vi "niRFUtil WFM Average (real wfm).vi"(0 "Waveform In":T2 {"y" min=0 max=127 format="%.2f"; "dx" format="%^.2e"; "x0" format="%^.2e"}, 5 "Average Mode":enum16{"Exponential", "Repeat"}(ring), 7 "Average Method":T1, 12 "Reset?":bool=TRUE, 13 "Initialize?":bool=TRUE) -> (4 "Average Out":T2 {"y" min=0 max=127 format="%.2f"; "dx" format="%^.2e"; "x0" format="%^.2e"})   [LabVIEW 2015, in "niRFUtil.lvlib"]
doc: "(c) Copyright 2006, National Instruments, Inc. This VI may not be duplicated, sold, or distributed without written consent from National Instruments."
uses:
  niRFUtil.lvlib
  Includes/niRFUtil INC Real Waveform.ctl
  Includes/niRFUtil INC Real Array.ctl
  Includes/niRFUtil INC Average Methods.ctl
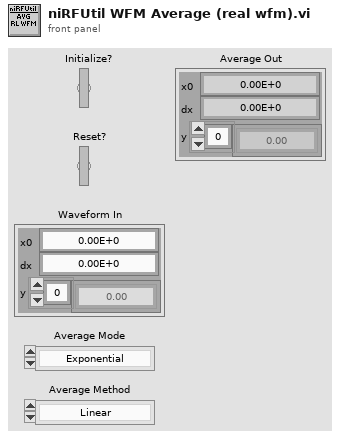
[diagram p1: front panel]
types:
  T1 = typedef "niRFUtil.lvlib/niRFUtil INC Average Methods.ctl" = enum16{"Linear", "Log", "Root", "Max", "Min", "MinMax"}
  T2 = typedef "niRFUtil.lvlib/niRFUtil INC Real Waveform.ctl" = cluster{"x0":dbl, "dx":dbl, "y":T3}
  T3 = typedef "niRFUtil.lvlib/niRFUtil INC Real Array.ctl" = sgl[]
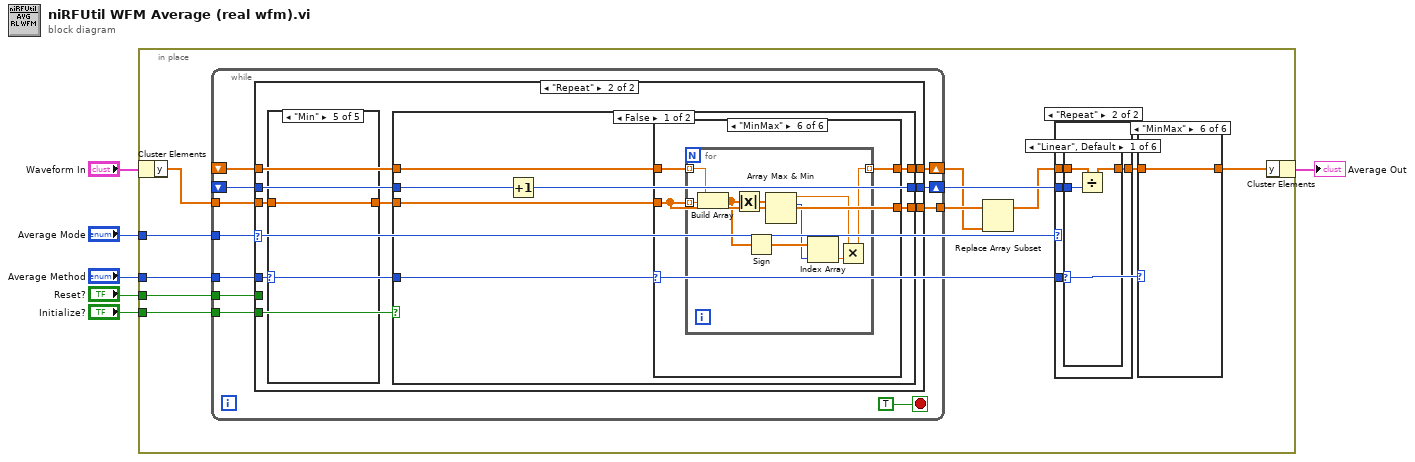
[diagram p0: block diagram]
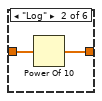
[diagram p3: hidden frame]
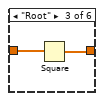
[diagram p4: hidden frame]
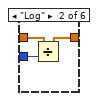
[diagram p8: hidden frame]
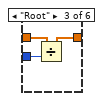
[diagram p9: hidden frame]
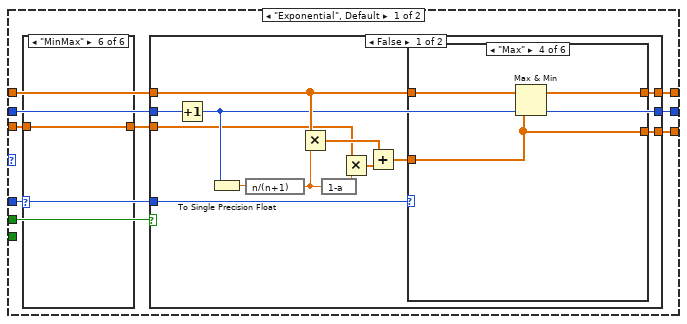
[diagram p13: hidden frame]
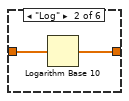
[diagram p15: hidden frame]
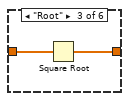
[diagram p16: hidden frame]
diagram:
  n1 = in-place {
    in-place-border: "Average Mode" -> [w16]
    in-place-border: "Average Method" -> [w15]
    in-place-border: "Reset?" -> [w14]
    in-place-border: "Initialize?" -> [w13]
    n2 = in-place-cluster #1("Waveform In") -> ("y"=w11:T3)
    n3 = while {
      shift-right: [w50] -> w8
      shift-left: _ -> [w47]
      tunnel: w16 -> [w52]
      tunnel: w14 -> [w51]
      tunnel: w11 -> [w49]
      shift-right: [w48] -> w17
      shift-left: _ -> [w46]
      tunnel: w15 -> [w45]
      tunnel: w13 -> [w44]
      tunnel: [w43] -> w9
      stop <- TRUE stop-if-true
      n4 = case shown="\"Repeat\"" w52 {
        tunnel: w51 -> [w59 _]
        tunnel: [w62 w115] -> w50
        tunnel: w49 -> [w57 w110]
        tunnel: [w58 w112] -> w48
        tunnel: w47 -> [w61 w114]
        tunnel: w46 -> [w60 w113]
        tunnel: w45 -> [w55 w108]
        tunnel: w44 -> [_ w111]
        tunnel: [w54 w107] -> w43
        frame "Exponential", Default {
          n5 = case shown="\"MinMax\"" w55 {
            tunnel: w57 -> [w63 w65 w67 w68 w69 w70]
            tunnel: [w63 w64 w66 w68 w69 w70] -> w56
            frame "Linear", Default {
            }
            frame "Log" {
              n6 = Logarithm Base 10(1:w65) -> (0:w64:T3)
            }
            frame "Root" {
              n7 = Square Root(x=w67) -> (sqrt(x)=w66:T3)
            }
            frame "Max" {
            }
            frame "Min" {
            }
            frame "MinMax" {
            }
          }
          n8 = case shown="False" w59 {
            tunnel: w56 -> [w72 w105]
            tunnel: [w78 w105] -> w62
            tunnel: w61 -> [w76 _]
            tunnel: w60 -> [w75 _]
            tunnel: [w74 1] -> w58
            tunnel: w55 -> [w73 _]
            tunnel: [w71 w105] -> w54
            frame False {
              n9 = Increment(x=w75) -> (x+1=w74:i32)
              n10 = To Single Precision Float(number=w74) -> (single precision float=w83:sgl)
              n11 = expression code="n/(n+1)"(w83) -> (w82:sgl)
              n12 = Multiply(x=w76, y=w82) -> (x*y=w79:T3)
              n13 = expression code="1-a"(w82) -> (w81:sgl)
              n14 = Multiply(x=w72, y=w81) -> (x*y=w80:T3)
              n15 = Add(x=w79, y=w80) -> (x+y=w77:T3)
              n16 = case shown="\"Max\"" w73 {
                tunnel: [w84 w85 w86 w88 w91 w94] -> w78
                tunnel: w77 -> [w84 w85 w86 w87 w90 w93]
                tunnel: w76 -> [_ _ _ w89 w92 w95]
                tunnel: [w84 w85 w86 w87 w90 w93] -> w71
                frame "Linear", Default {
                }
                frame "Log" {
                }
                frame "Root" {
                }
                frame "Max" {
                  n17 = Max & Min(x=w89, y=w87) -> (max(x,y)=w88:T3)  [unwired: 1 out]
                }
                frame "Min" {
                  n18 = Max & Min(x=w92, y=w90) -> (min(x,y)=w91:T3)  [unwired: 1 out]
                }
                frame "MinMax" {
                  n19 = for {
                    tunnel: w95 -> [w101] mode=indexing
                    tunnel: [w100] -> w94 mode=indexing
                    tunnel: w93 -> [w98] mode=indexing
                    n20 = Build Array(w101, w98) -> (w104:sgl[])
                    n21 = Absolute Value(x=w104) -> (abs(x)=w99:sgl[])
                    n22 = Sign(1:w104) -> (0:w103:sgl[])
                    n23 = Array Max & Min(array=w99) -> (max value=w97:sgl, max index (indices)=w96:i32)  [unwired: 2 out]
                    n24 = Index Array(array=w103, index=w96) -> (element=w102:sgl)
                    n25 = Multiply(x=w97, y=w102) -> (x*y=w100:sgl)
                  }
                }
              }
            }
            frame True {
            }
          }
        }
        frame "Repeat" {
          n26 = case shown="\"Min\"" w108 {
            tunnel: w110 -> [w116 w118 w120 w121 w122]
            tunnel: [w116 w117 w119 w121 w122] -> w109
            frame "Linear", Default {
            }
            frame "Log" {
              n27 = Logarithm Base 10(1:w118) -> (0:w117:T3)
            }
            frame "Root" {
              n28 = Square Root(x=w120) -> (sqrt(x)=w119:T3)
            }
            frame "Max" {
            }
            frame "Min" {
            }
          }
          n29 = case shown="False" w111 {
            tunnel: w109 -> [w124 w157]
            tunnel: [w129 w157] -> w115
            tunnel: w114 -> [w128 _]
            tunnel: w113 -> [w127 _]
            tunnel: [w126 1] -> w112
            tunnel: w108 -> [w125 _]
            tunnel: [w123 w157] -> w107
            frame False {
              n30 = Increment(x=w127) -> (x+1=w126:i32)
              n31 = case shown="\"MinMax\"" w125 {
                tunnel: [w131 w134 w137 w140 w143 w146] -> w129
                tunnel: w128 -> [w132 w135 w138 w141 w144 w147]
                tunnel: w124 -> [w130 w133 w136 w139 w142 w145]
                tunnel: [w130 w133 w136 w139 w142 w145] -> w123
                frame "Linear", Default {
                  n32 = Add(x=w132, y=w130) -> (x+y=w131:T3)
                }
                frame "Log" {
                  n33 = Add(x=w135, y=w133) -> (x+y=w134:T3)
                }
                frame "Root" {
                  n34 = Add(x=w138, y=w136) -> (x+y=w137:T3)
                }
                frame "Max" {
                  n35 = Max & Min(x=w141, y=w139) -> (max(x,y)=w140:T3)  [unwired: 1 out]
                }
                frame "Min" {
                  n36 = Max & Min(x=w144, y=w142) -> (min(x,y)=w143:T3)  [unwired: 1 out]
                }
                frame "MinMax" {
                  n37 = for {
                    tunnel: w147 -> [w153] mode=indexing
                    tunnel: [w152] -> w146 mode=indexing
                    tunnel: w145 -> [w150] mode=indexing
                    n38 = Build Array(w153, w150) -> (w156:sgl[])
                    n39 = Absolute Value(x=w156) -> (abs(x)=w151:sgl[])
                    n40 = Sign(1:w156) -> (0:w155:sgl[])
                    n41 = Array Max & Min(array=w151) -> (max value=w149:sgl, max index (indices)=w148:i32)  [unwired: 2 out]
                    n42 = Index Array(array=w155, index=w148) -> (element=w154:sgl)
                    n43 = Multiply(x=w149, y=w154) -> (x*y=w152:sgl)
                  }
                }
              }
            }
            frame True {
            }
          }
        }
      }
    }
    n44 = Replace Array Subset(array=w9, new element=w8) -> (w7:T3)  [unwired: 1 in]
    n45 = case shown="\"Repeat\"" w16 {
      tunnel: [w26 w28] -> w12
      tunnel: w7 -> [w26 w29]
      tunnel: w17 -> [_ w30]
      tunnel: w15 -> [_ w27]
      frame "Exponential", Default {
      }
      frame "Repeat" {
        n46 = case shown="\"Linear\", Default" w27 {
          tunnel: w30 -> [w33 w36 w39 _ _ _]
          tunnel: w29 -> [w32 w35 w38 w40 w41 w42]
          tunnel: [w31 w34 w37 w40 w41 w42] -> w28
          frame "Linear", Default {
            n47 = Divide(x=w32, y=w33) -> (x/y=w31:T3)
          }
          frame "Log" {
            n48 = Divide(x=w35, y=w36) -> (x/y=w34:T3)
          }
          frame "Root" {
            n49 = Divide(x=w38, y=w39) -> (x/y=w37:T3)
          }
          frame "Max" {
          }
          frame "Min" {
          }
          frame "MinMax" {
          }
        }
      }
    }
    n50 = case shown="\"MinMax\"" w15 {
      tunnel: w12 -> [w18 w20 w22 w23 w24 w25]
      tunnel: [w18 w19 w21 w23 w24 w25] -> w10
      frame "Linear", Default {
      }
      frame "Log" {
        n51 = Power Of 10(x=w20) -> (10^x=w19:T3)
      }
      frame "Root" {
        n52 = Square(x=w22) -> (x^2=w21:T3)
      }
      frame "Max" {
      }
      frame "Min" {
      }
      frame "MinMax" {
      }
    }
    n53 = in-place-cluster #1("y"=w10) -> (→"Average Out":T2)
  }
